vi "ScanFromString.vi"() -> ()   [LabVIEW 2019]
panel:
  out "String":string
  in  "salary":u16
  in  "age":u8
  in  "name":string
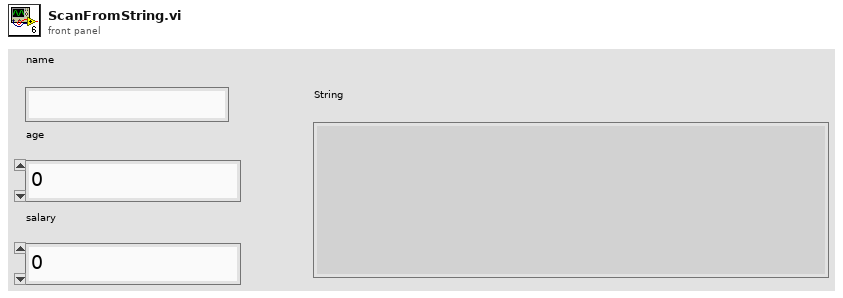
[diagram p1: front panel]
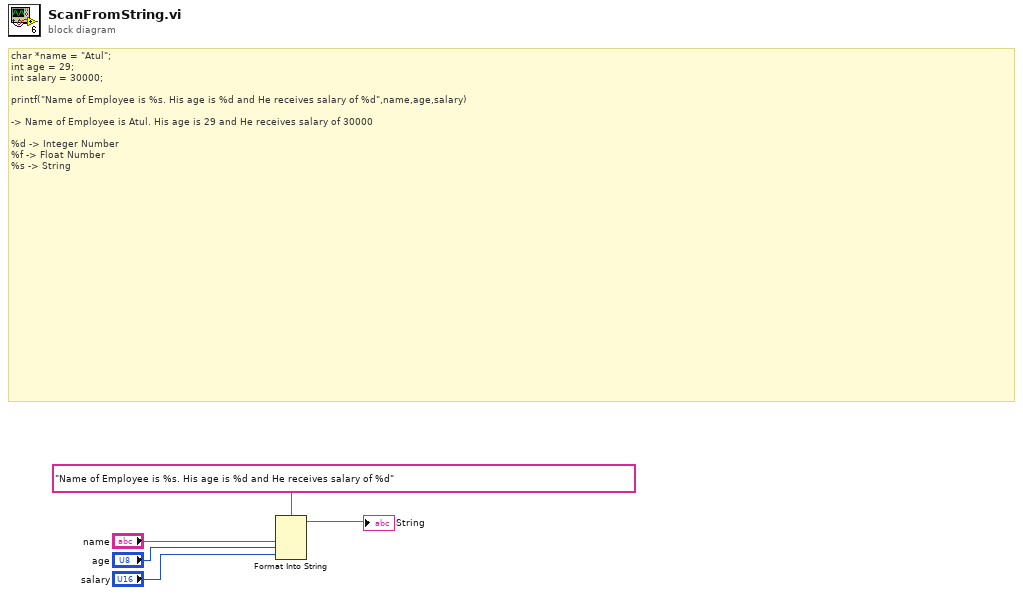
[diagram p0: block diagram]
diagram:
  # "char *name = \"Atul\"; \nint age = 29;\nint salary = 30000;\n\nprintf(\"Name of Employee is %s. His age is %d and He receives salary of %d\",name,age,salary)\n\n-> Name of Employee is Atul. His age is 29 and He receives salary of 30000\n\n%d -> Integer Number\n%f -> Float Number\n%s -> String"
  n1 = Format Into String(format string="Name of Employee is %s. His age is %d and He receives salary of %d", "name", "age", "salary") -> (resulting string=→"String":string)  [unwired: 2 in, 1 out]
